vi "End Events.vi"(1 "Event Registration Refnum in":refnum<event-registration>, 2 "output cluster":T1) -> ()   [LabVIEW 2021]
uses:
  event cluster.ctl
panel:
  out "error out":errorcluster
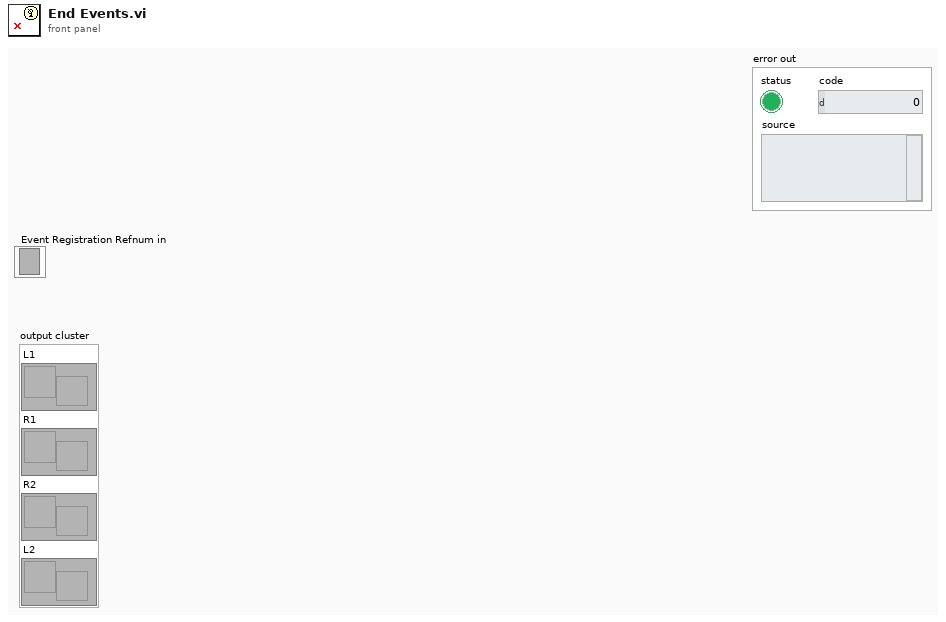
[diagram p1: front panel]
types:
  T1 = typedef "event cluster.ctl" = cluster{"L1":refnum<user-event>, "R1":refnum<user-event>, "R2":refnum<user-event>, "L2":refnum<user-event>}
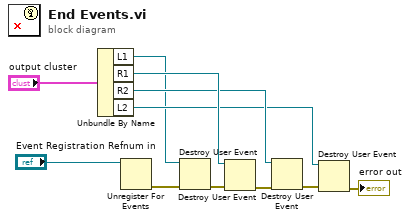
[diagram p0: block diagram]
diagram:
  n1 = Unbundle By Name("output cluster") -> ("L1"=w5:refnum<user-event>, "R1"=w11:refnum<user-event>, "R2"=w10:refnum<user-event>, "L2"=w9:refnum<user-event>)
  n2 = Unregister For Events(event registration refnum="Event Registration Refnum in") -> (error out=w3:errorcluster)  [unwired: 1 in]
  n3 = Destroy User Event(user event=w5, error in=w3) -> (error out=w6:errorcluster)
  n4 = Destroy User Event(user event=w11, error in=w6) -> (error out=w7:errorcluster)
  n5 = Destroy User Event(user event=w10, error in=w7) -> (error out=w8:errorcluster)
  n6 = Destroy User Event(user event=w9, error in=w8) -> (error out=→"error out":errorcluster)
